vi "Control Resistance.vi"(8 "error in (no error)":errorcluster, 10 "resistance params":T2, 11 "Refnum in":T1) -> (0 "error out":errorcluster)   [LabVIEW 2017, in "NI 272x Resistive Simulation Custom Device Engine.lvlib"]
uses:
  NI 272x Resistive Simulation Custom Device Engine.lvlib
  resistance params.ctl
  <vilib>/NI/NIVS Inline Async API/_Data Access Engine/Data Access Engine/Types/Write.DVR.ctl
  <vilib>/NI/NIVS Inline Async API/_Data Access Engine/Access Type Classes/Write/Write.lvclass
  <vilib>/NI/NIVS Inline Async API/_Data Access Engine/Data Access Engine/Types/Read.DVR.ctl
  <vilib>/NI/NIVS Inline Async API/_Data Access Engine/Access Type Classes/Read/Read.lvclass
  Controls/Compiled HW Channel.ctl
  Controls/Channel Mode.ctl
  <instrlib>/ni272xReferenceVIs/ni272xReferenceVIs.llb/ni272x Callendar-Van Dusen RTD Parameters.ctl
  <instrlib>/ni272xReferenceVIs/ni272xReferenceVIs.llb/ni272x Reference.ctl
  <vilib>/NI/NIVS Inline Async API/_Data Access Engine/Access Type Classes/Read/Read.lvclass/Read.ctl
  <vilib>/NI/NIVS Inline Async API/_Data Access Engine/Access Type Classes/Write/Write.lvclass/Write.ctl
  <vilib>/NI/NIVS Inline Async API/_Data Access Engine/Data Access Engine/Methods/Read.Data.Detect.vi
  <vilib>/NI/NIVS Inline Async API/_Data Access Engine/Data Access Engine/Methods/Write.Data.Buffer.vi
  <vilib>/NI/NIVS Inline Async API/_Data Access Engine/Data Access Engine/Methods/Write.Data.Commit.vi
  <vilib>/NI/NIVS Inline Async API/_Data Access Engine/Access Type Classes/Read/Read.ProcessData.Detect.vi
  <vilib>/NI/NIVS Inline Async API/_Data Access Engine/Access Type Classes/Write/Write.Buffer.vi
  <vilib>/NI/NIVS Inline Async API/_Data Access Engine/Access Type Classes/Write/Write.Commit.vi
  <vilib>/NI/NIVS Inline Async API/_Data Access Engine/Data Access Engine/Data Access Engine.lvclass
  NI 272x Resistive Simulation Custom Device Shared.lvlib
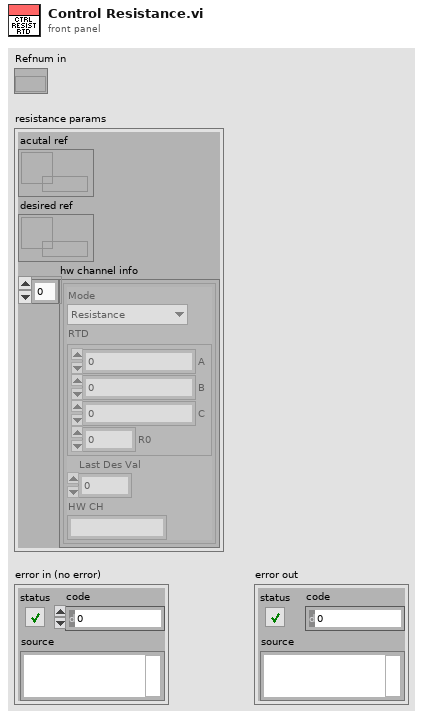
[diagram p1: front panel]
types:
  T1 = typedef "ni272x Reference.ctl" = refnum<k20>
  T2 = typedef "NI 272x Resistive Simulation Custom Device Engine.lvlib/resistance params.ctl" = cluster{"acutal ref":T3, "desired ref":T4, "hw channel info":T5[]}
  T3 = typedef "Data Access Engine.lvlib/Data Access Engine.lvclass/Write.DVR.ctl" = refnum<data-value>
  T4 = typedef "Data Access Engine.lvlib/Data Access Engine.lvclass/Read.DVR.ctl" = refnum<data-value>
  T5 = typedef "NI 272x Resistive Simulation Custom Device Shared.lvlib/Compiled HW Channel.ctl" = cluster{"Mode":T6, "RTD":T7, "Last Des Val":dbl, "HW CH":string}
  T6 = typedef "NI 272x Resistive Simulation Custom Device Shared.lvlib/Channel Mode.ctl" = enum16{"Resistance", "RTD Temperature"}
  T7 = typedef "ni272x Callendar-Van Dusen RTD Parameters.ctl" = cluster{"A":dbl, "B":dbl, "C":dbl, "R0":dbl}
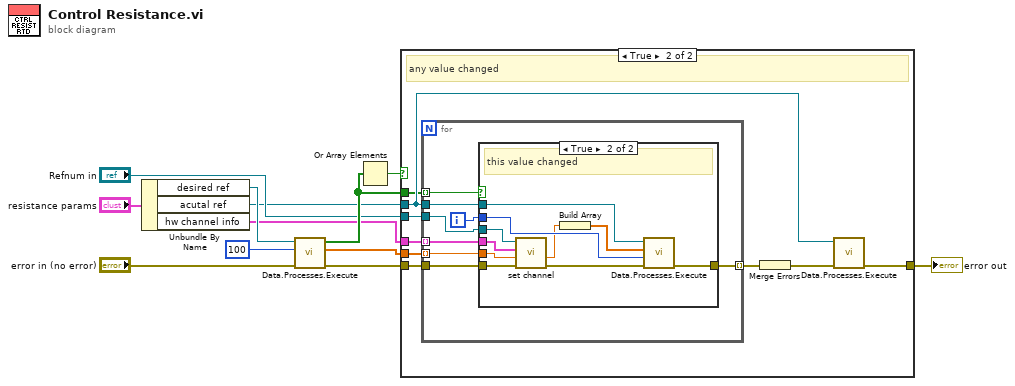
[diagram p0: block diagram]
diagram:
  n1 = Unbundle By Name("resistance params") -> ("desired ref"=w3:T4, "acutal ref"=w2:T3, "hw channel info"=w1:T5[])
  n2 = call-poly <vilib>:"Data.Processes.Execute.vi"("error in (no error)"="error in (no error)", "timeout ms"=100, "Ref"=w3) -> ("error out"=w10:errorcluster, "Values"=w8:dbl[], "Detect?"=w11:bool[])  [unwired: 5 in, 1 out]
  n3 = Or Array Elements(Boolean array=w11) -> (logical OR=w12:bool)
  n4 = case shown="True" w12 {
    tunnel: [w13 w22] -> w6
    tunnel: w8 -> [_ w21]
    tunnel: "Refnum in" -> [_ w20]
    tunnel: w1 -> [_ w19]
    tunnel: w10 -> [w13 w17]
    tunnel: w2 -> [_ w15]
    tunnel: w11 -> [_ w14]
    frame False {
      # "no value change"
    }
    frame True {
      # "any value changed"
      n5 = for {
        tunnel: w14 -> [w29] mode=indexing
        tunnel: w21 -> [w27] mode=indexing
        tunnel: w20 -> [w30]
        tunnel: w19 -> [w28] mode=indexing
        tunnel: [w26] -> w18 mode=indexing
        tunnel: w17 -> [w25]
        tunnel: w15 -> [w24]
        i -> [w23]
        n6 = case shown="True" w29 {
          tunnel: w30 -> [_ w41]
          tunnel: w28 -> [_ w40]
          tunnel: w27 -> [_ w39]
          tunnel: [w31 w34] -> w26
          tunnel: w25 -> [w31 w38]
          tunnel: w24 -> [_ w37]
          tunnel: w23 -> [_ w36]
          frame False {
            # "this value did not change"
          }
          frame True {
            # "this value changed"
            n7 = call "set channel.vi"("error in (no error)"=w38, "Channel Data Reference"=w39, "HW Chn"=w40, "Refnum in"=w41) -> ("error out"=w35:errorcluster, "coerced resistance (ohms)"=w33:dbl)  [unwired: 6 in]
            n8 = Build Array(w33) -> (w32:dbl[])
            n9 = call-poly <vilib>:"Data.Processes.Execute.vi"("error in (no error)"=w35, "Offset"=w36, "Values"=w32, "Ref"=w37) -> ("error out"=w34:errorcluster)  [unwired: 7 in]
          }
        }
      }
      n10 = Merge Errors(w18) -> (w16:errorcluster)
      n11 = call-poly <vilib>:"Data.Processes.Execute.vi"("error in (no error)"=w16, "Ref"=w15) -> ("error out"=w22:errorcluster)  [unwired: 9 in]
    }
  }
  "error out" <- w6
